vi "Microscopy.Circular Buffer (BRAM)_Array_Multi-Channel.vi"(7 "Buffer Pointers":T4, 8 "Input Valid":bool, 9 "Read Data?":bool, 10 "Acquisition Status In":T1={"Reset"=FALSE, "Acquisition Engine Start (Arm)"=FALSE, "Current State"=enum."Acquire Pre-Trigger Samples", "Trig Offset"=0, "Points Unread"=0, "Points Acquired"=0, "Records Done"=0, "Start of Read"=FALSE, "End of Read"=FALSE, "Start of Record"=FALSE, "End of Record"=FALSE, "Ready for Ref Trig"=FALSE, "In Reset?"=FALSE}, 11 "Input Write Data":T3=[0, 0, 0, 0]) -> (0 "Output Valid":bool, 2 "Acquisition Status Out":T1={"Reset"=FALSE, "Acquisition Engine Start (Arm)"=FALSE, "Current State"=enum."Acquire Pre-Trigger Samples", "Trig Offset"=0, "Points Unread"=0, "Points Acquired"=0, "Records Done"=0, "Start of Read"=FALSE, "End of Read"=FALSE, "Start of Record"=FALSE, "End of Record"=FALSE, "Ready for Ref Trig"=FALSE, "In Reset?"=FALSE}, 3 "Output Write Data":T3)   [LabVIEW 2012]
doc: "This VI maintains a circular buffer with user configurable buffer size.\nMaximum Buffer Size = 4096 (U32) elements\n\n<b> Delay = 1 Tick </b>"
uses:
  Buffer Parameters.ctl
  Multi-Channel Analog Input Data.ctl
  Acquisition Status.ctl
  Acquisition Engine State.ctl
  <vilib>/rvi/DataTransferAndStorage/Container/Common/niFpgaContainerMetaDataKey.ctl
  <vilib>/rvi/DataTransferAndStorage/Container/Common/niFpgaContainerState.ctl
  <vilib>/rvi/DataTransferAndStorage/Container/Common/niFpgaDataTypeControl.ctl
  <vilib>/rvi/DataTransferAndStorage/Container/Common/niFpgaContainerImplementationControl.ctl
  <vilib>/rvi/DataTransferAndStorage/Container/Common/niFpgaContainerArbitrationOptionsControl.ctl
  <vilib>/rvi/DataTransferAndStorage/Container/Common/niFpgaTransferTypeControl.ctl
  <vilib>/rvi/DataTransferAndStorage/Container/Common/niFpgaContainerInitializationParameters.ctl
  <vilib>/rvi/Memory/Memory_Types/niFpgaMemoryInterfaceConfiguration.ctl
  <vilib>/rvi/FIFO/Fifo_Types/niFpgaFifoControlLogicControl.ctl
  <vilib>/rvi/DataTransferAndStorage/Container/Common/niFpgaContainerGetUniqueNameForEmu.vi
  <vilib>/rvi/DataTransferAndStorage/Container/Common/niFpgaContainerSetEmuInfo.vi
  <vilib>/rvi/eio/common/nirviEmuReportErrorAndStop.vi
  <vilib>/rvi/Memory/Memory_Emulation/niFpgaMemoryEmulationCacheClearOnFirstRun.vi
  <vilib>/rvi/Memory/Memory_Emulation/nirvimemoryEmulationManagerCache_MakeExclusive.vi
  <vilib>/rvi/Memory/Memory_Emulation/niFpgaMemoryEmulationValidateCache.vi
  <vilib>/rvi/Memory/Memory_Emulation/nirvimemoryEmulationManagerCache_ReleaseExclusive.vi
  <vilib>/rvi/Memory/Memory_Emulation/nirvimemoryEmulationManagerCache_InsertValue.vi
  <vilib>/Utility/error.llb/Clear Errors.vi
  <vilib>/rvi/Memory/Memory_Emulation/nirvimemoryEmulationManagerCache_GetValue.vi
  <vilib>/rvi/Emulation/niFpgaSctlEmulationGetInTimedLoop.vi
  <vilib>/rvi/Memory/Memory_Emulation/nirvimemoryEmulationManagerCache_SetValue.vi
  <vilib>/rvi/Emulation/niFpgaSctlEmulationResourceMgr.vi
  <vilib>/rvi/LocalResourceManager/LocalResourceManager.xnode
  <vilib>/rvi/DataTransferAndStorage/Container/XNode/niFpgaContainer.xnode
  <vilib>/rvi/Memory/Memory_Emulation/nirvimemoryEmulation.vi
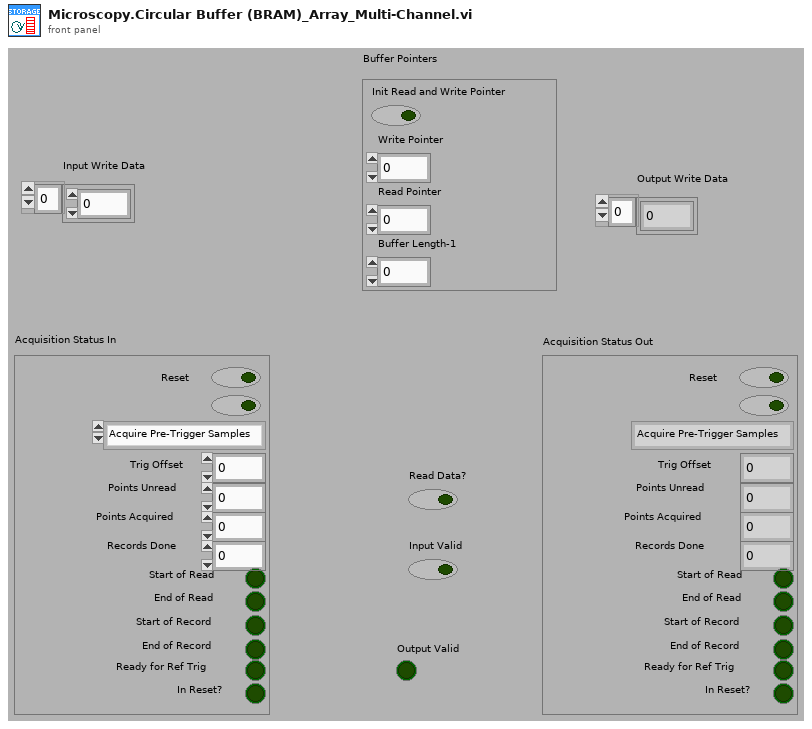
[diagram p1: front panel]
types:
  T1 = typedef "Acquisition Status.ctl" = cluster{"Reset":bool, "Acquisition Engine Start (Arm)":bool, "Current State":T2, "Trig Offset":u8, "Points Unread":u16, "Points Acquired":u16, "Records Done":u16, "Start of Read":bool, "End of Read":bool, "Start of Record":bool, "End of Record":bool, "Ready for Ref Trig":bool, "In Reset?":bool}
  T2 = typedef "Acquisition Engine State.ctl" = enum8{"Idle", "Arm Acquisition Engine", "Acquire Pre-Trigger Samples", "Wait for Trigger", "Acquisition Hold Off Time", "Read Data from Buffer", "Check Records Done?", "Re-Arm State", "Flush Available Data"}
  T3 = typedef "Multi-Channel Analog Input Data.ctl" = i16[]
  T4 = typedef "Buffer Parameters.ctl" = cluster{"Init Read and Write Pointer":bool, "Write Pointer":u16, "Read Pointer":u16, "Buffer Length-1":u16}
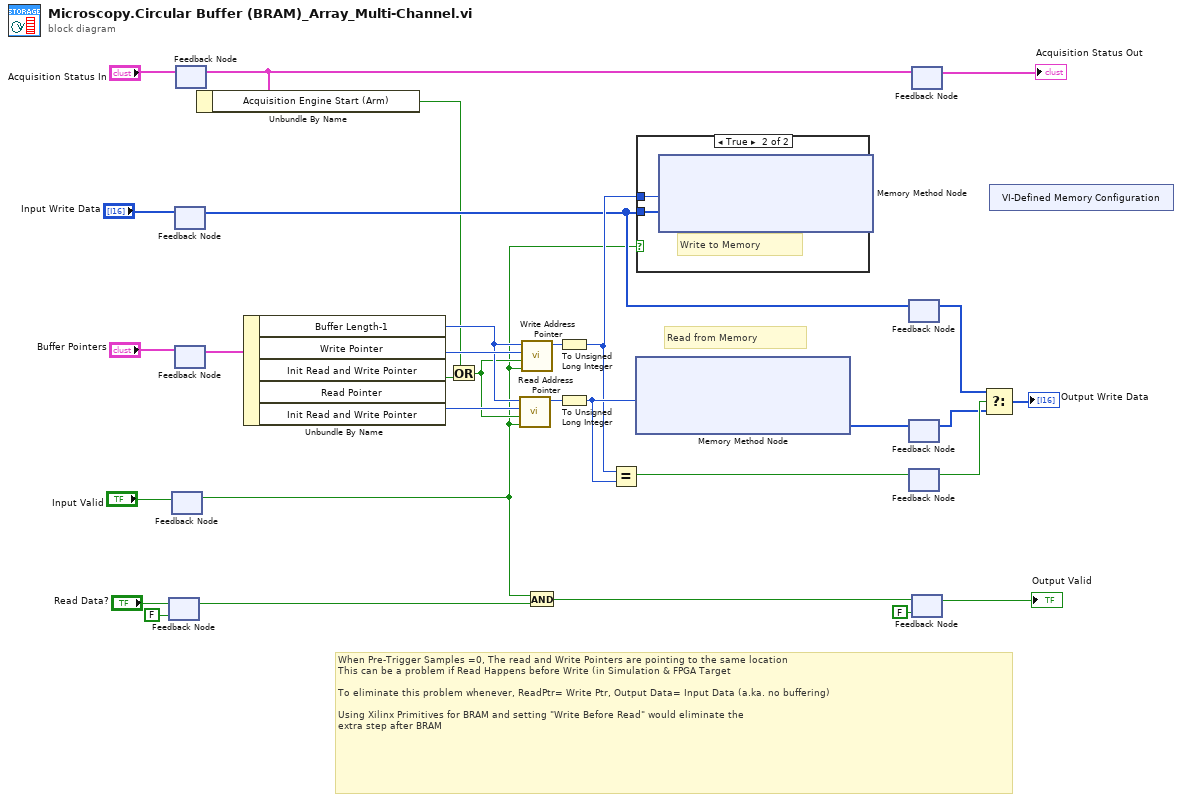
[diagram p0: block diagram]
diagram:
  # "When Pre-Trigger Samples =0, The read and Write Pointers are pointing to the same location\nThis can be a problem if Read Happens before Write (in Simulation & FPGA Target\n\nTo eliminate this problem whenever, ReadPtr= Write Ptr, Output Data= Input Data (a.ka. no buffering)\n\nUsing Xilinx Primitives for BRAM and setting \"Write Before Read\" would eliminate the\nextra step after BRAM"
  # "Read from Memory"
  n1 = feedback-in #1("Read Data?") -> ()
  n2 = feedback #1(FALSE ("Read Data?")) -> (w2:bool)
  n3 = feedback #2() -> (w3:bool)  [unwired: 1 in]
  n4 = feedback-in #2("Input Valid") -> ()
  n5 = feedback #3() -> (w15:T3)  [unwired: 1 in]
  n6 = feedback-in #3("Input Write Data") -> ()
  n7 = feedback #4() -> (w30:T4)  [unwired: 1 in]
  n8 = feedback-in #4("Buffer Pointers") -> ()
  n9 = feedback #5() -> (w9:T1)  [unwired: 1 in]
  n10 = feedback-in #5("Acquisition Status In") -> ()
  n11 = Unbundle By Name(w9) -> ("Acquisition Engine Start (Arm)"=w7:bool)
  n12 = Unbundle By Name(w30) -> ("Buffer Length-1"=w22:u16, "Write Pointer"=w24:u16, "Init Read and Write Pointer"=w8:bool, "Read Pointer"=w23:u16)  [unwired: 1 out]
  n13 = Or(x=w7, y=w8) -> (x .or. y?=w6:bool)
  n14 = call "Read Address Pointer.vi"("INC?"=w3, "Load?"=w6, "Load Value"=w23, "rollover"=w22) -> ("count"=w5:u16)  [unwired: 7 in]
  n15 = call "Write Address Pointer.vi"("INC?"=w3, "Load?"=w6, "Load Value"=w24, "rollover"=w22) -> ("count"=w4:u16)  [unwired: 7 in]
  n16 = And(x=w3, y=w2) -> (x .and. y?=w1:bool)
  n17 = To Unsigned Long Integer(number=w4) -> (unsigned 32bit integer=w18:u32)
  n18 = To Unsigned Long Integer(number=w5) -> (unsigned 32bit integer=w21:u32)
  n19 = Equal?(x=w18, y=w21) -> (x = y?=w19:bool)
  n20 = xnode ("Memory Method Node")("Address"=w21) -> ("Data"=w31:i16[])  [unwired: 1 in, 1 out]
  n21 = case shown="True" w3 {
    tunnel: w15 -> [_ w33]
    tunnel: w18 -> [_ w32]
    frame False {
    }
    frame True {
      # "Write to Memory"
      n22 = xnode ("Memory Method Node")("Address"=w32, "Data"=w33) -> ()  [unwired: 1 in, 1 out]
    }
  }
  n23 = feedback #6() -> (w17:T3)  [unwired: 1 in]
  n24 = feedback-in #6(w15) -> ()
  n25 = feedback #7() -> (w16:i16[])  [unwired: 1 in]
  n26 = feedback-in #7(w31) -> ()
  n27 = feedback #8() -> (w20:bool)  [unwired: 1 in]
  n28 = feedback-in #8(w19) -> ()
  n29 = feedback #9() -> (→"Acquisition Status Out":T1)  [unwired: 1 in]
  n30 = feedback-in #9(w9) -> ()
  n31 = feedback #10(FALSE ("Retrieve Data")) -> (→"Output Valid":bool)
  n32 = feedback-in #10(w1) -> ()
  n33 = Select(t=w17, s=w20, f=w16) -> (s? t:f=→"Output Write Data":T3)
  n34 = xnode "VI-Defined Memory Configuration"() -> ()  [unwired: 1 out]
